vi "TopLevelRelativeToAbsolutePath.vi"(8 "error in (no error)":errorcluster, 11 "Path Relative to Top Level VI":path) -> (0 "error out":errorcluster, 3 "Absolute path":path)   [LabVIEW 2018]
doc: "If the input path is a relative path, this VI returns the absolute path if the input path is relative to the location of the current top-level VI. Otherwise the VI returns the input path."
panel:
  # "LVHDF5 Example VI\nCopyright (c) 2014 UPVI, LLC\nwww.upvi.net\n\nThis VI is exempt from the LVHDF5 license and may be freely copied, modified, distributed or incorporated into other applications."
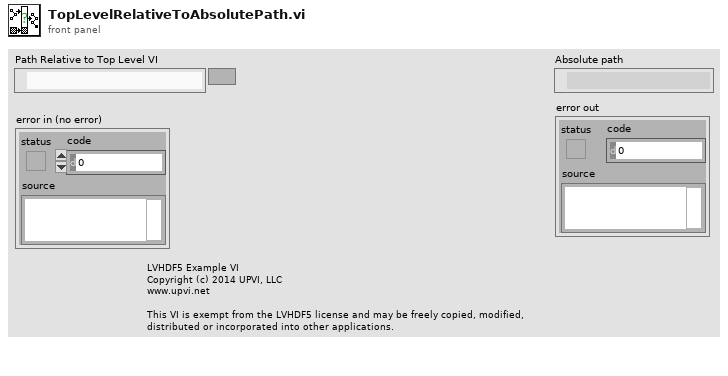
[diagram p1: front panel]
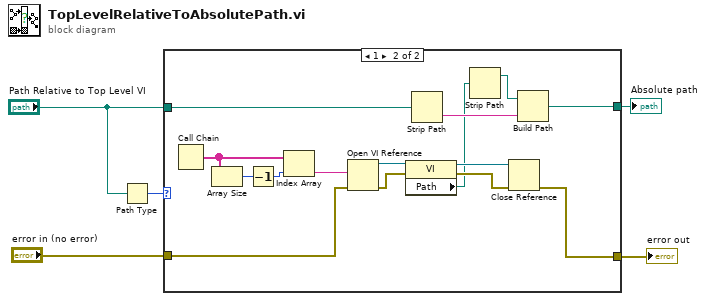
[diagram p0: block diagram]
diagram:
  n1 = Path Type(1:"Path Relative to Top Level VI") -> (0:w5:i16)
  n2 = case shown="1" w5 {
    tunnel: "error in (no error)" -> [w7 w14]
    tunnel: "Path Relative to Top Level VI" -> [w6 w13]
    tunnel: [w6 w11] -> w1
    tunnel: [w7 w10] -> w2
    frame 0, Default {
    }
    frame 1 {
      n3 = Call Chain() -> (call chain=w15:string[])
      n4 = Array Size(array=w15) -> (size(s)=w16:i32)
      n5 = Decrement(x=w16) -> (x-1=w17:i32)
      n6 = Index Array(array=w15, index=w17) -> (element=w18:string)
      n7 = Open VI Reference(vi path=w18, error in (no error)=w14) -> (vi reference=w19:refnum<vi>, error out=w20:errorcluster)  [unwired: 4 in]
      n8 = property class="VI"(reference=w19, error in=w20) -> (reference out=w21:refnum<vi>, error out=w22:errorcluster, "Path"=w8:path)
      n9 = Strip Path(path=w13) -> (name=w12:string)  [unwired: 1 out]
      n10 = Strip Path(path=w8) -> (stripped path=w9:path)  [unwired: 1 out]
      n11 = Close Reference(reference=w21, error in (no error)=w22) -> (error out=w10:errorcluster)
      n12 = Build Path(base path=w9, name or relative path=w12) -> (appended path=w11:path)
    }
  }
  "error out" <- w2
  "Absolute path" <- w1
